vi "0MAIN _v2.vi"() -> ()   [LabVIEW 2014]
uses:
  <vilib>/Instr/_visa.llb/VISA Configure Serial Port (Instr).vi
  <vilib>/Instr/_visa.llb/VISA Open Access Mode.ctl
panel:
  out "OSL":bool
  out "Ошибка файла":errorcluster
  out "firstL":bool
  out "LN":bool
  out "WFL":bool
  out "SPL":bool
  out "umax":dbl
  out "umin":dbl
  out "fmax":dbl
  out "fmin":dbl
  out "FCD":bool
  out "LF2":bool
  out "LF1":bool
  out "В лог":string
  out "Строит":bool
  out "Ошибка temp":errorcluster
  out "Читает":bool
  out "Время старта":string
  out "Ошибка лога":errorcluster
  out "Файл данных":refnum<file>
  out "Файл журнала":refnum<file>
  in  "Управление":enum32{"Измерения", "График", "Настройки"}(tab)
  in  "SREP":bool
  in  "SR":bool
  in  "SP":T1 caption="Программа измерений" {"Шаг" format="%#_3g"; "Fкон" format="%#_3g"; "Fнач" format="%#_3g"}
  in  "Автограф":bool
  in  "Расчет графика":bool
  in  "TOF":bool
  in  "Частота метки 2":bool
  in  "Сохранение данных":bool
  in  "Очистка буфера":bool
  in  "Чтение данных":bool
  in  "Установить":string
  in  "Отправка":bool
  out "Данные с МК":string
  in  "Частота метки":bool
  in  "Выход":bool
  in  "Очистка массива":bool
  out "Сигналы":dbl[][](array[numeric]) caption="Сигнал Y, В" format="%#_3g"
  out "Метки":dbl[][](array[numeric]) caption="Метки:\nX (В)          Х (ГГц)"
  in  "SS":bool
  out "График":T2(graph)
  in  "Путь к файлу данных":path
  in  "Путь к логу":path
  in  "Логирование":bool
  out "Ошибка":T3
  in  "Порт":refnum<visa-resource-name>
  in  "Скорость передачи (9600)":u32=9600
  in  "Символ окончания (\\n)":u8=10 format="%.0x"
  in  "Режим доступа":T4 items=["VISA Defaults"=0, "Exclusive Lock"=1, "Load Configured Settings"=4]
  in  "Бит данных (8)":u8=8 format="%.0x"
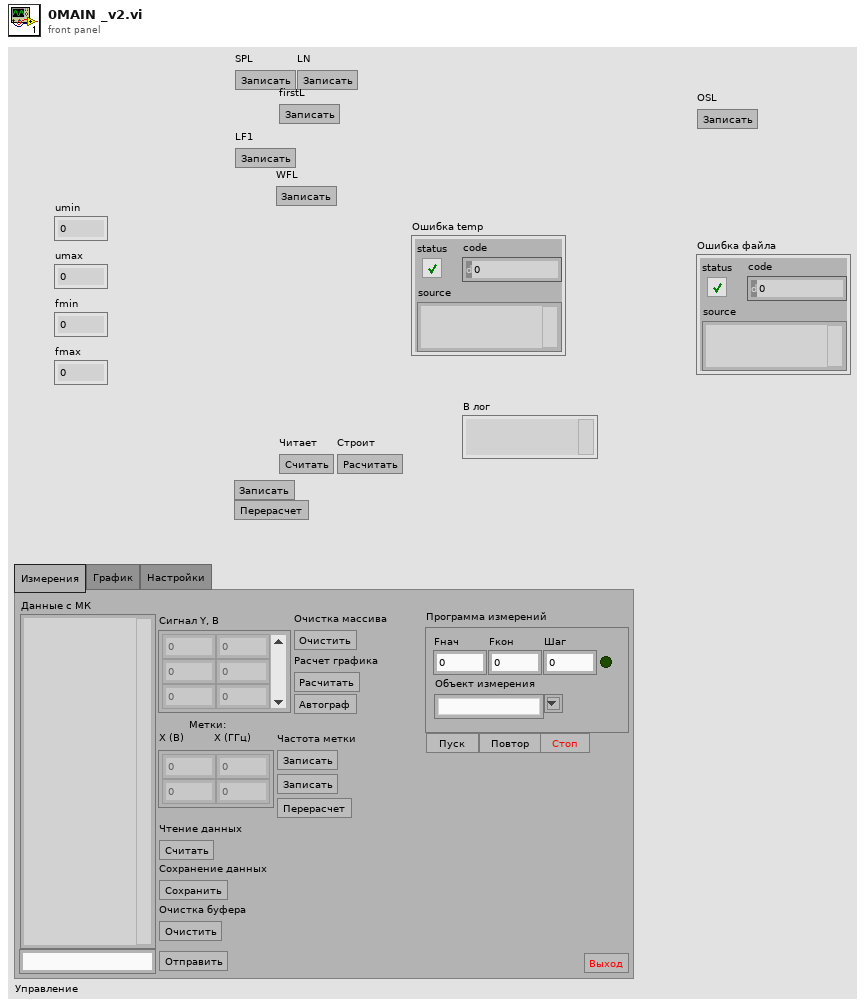
[diagram p1: front panel]
types:
  T1 = cluster{"Fнач":dbl, "Fкон":dbl, "Шаг":dbl, "ISR":bool, "ux":dbl, "i":u64, "n":u64, "MT":string}
  T2 = cluster{"Развертка X (В)":dbl[], "Сигнал Y (В)":dbl[]}
  T3 = cluster{"Статус":bool, "Код":i32, "Источник":string}
  T4 = typedef "VISA Open Access Mode.ctl" = u32
  T5 = enum16{"open", "replace", "create", "open or create", "replace or create", "replace or create with confirmation"}
  T6 = typedef "NI_Matrix.lvlib/RealMatrix.ctl" = dbl[][]
  T7 = enum32{"Измерения", "График", "Настройки", "Справка"}
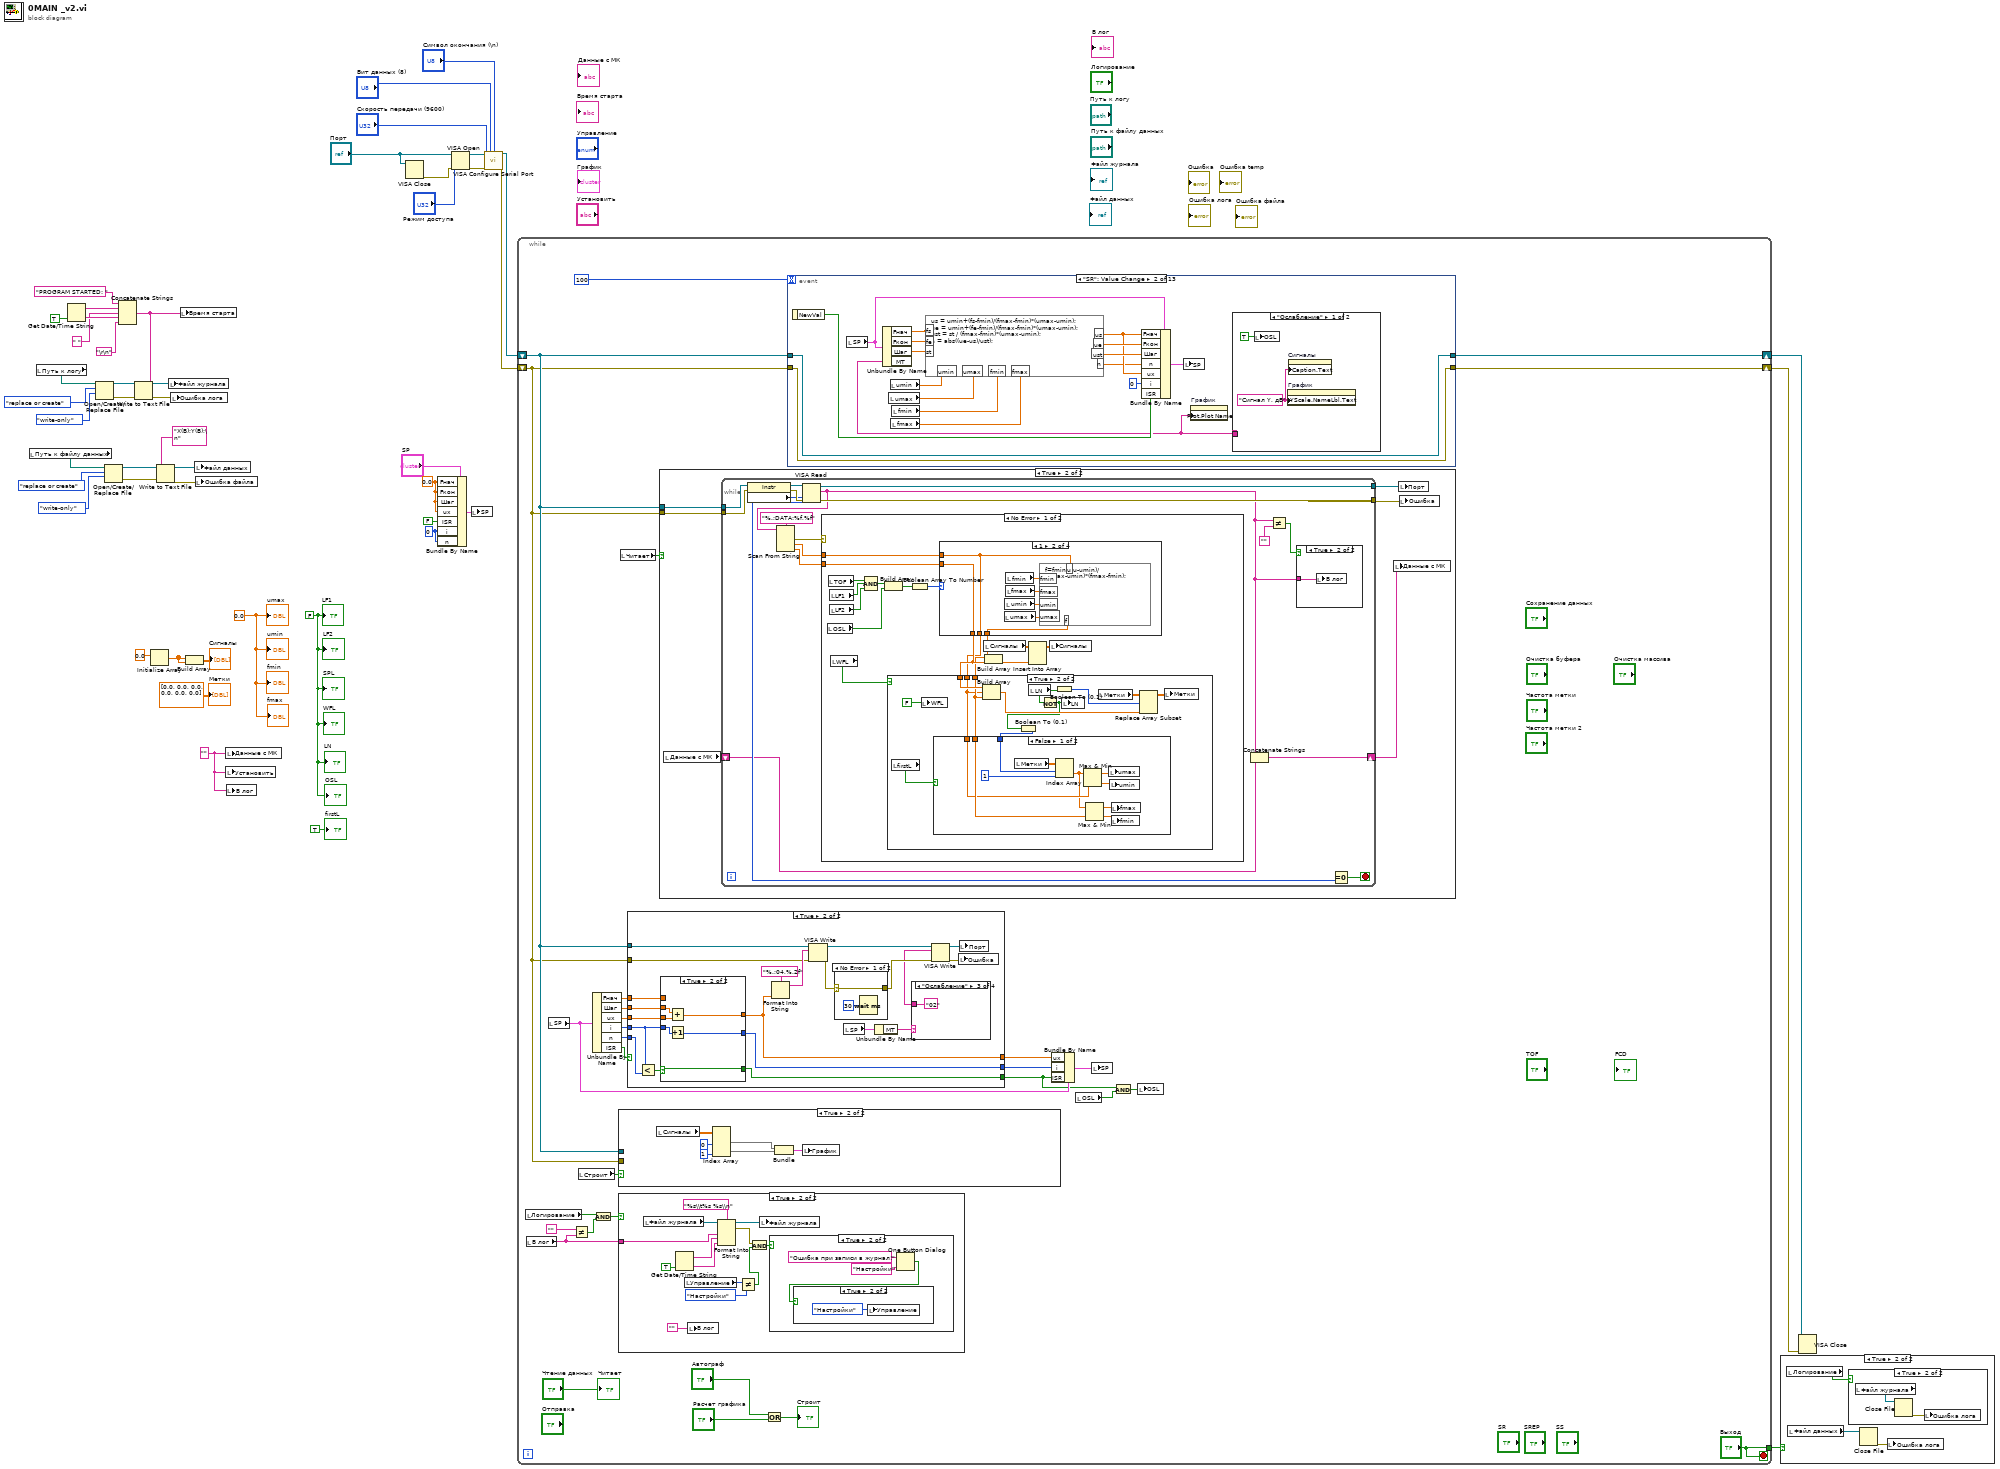
[diagram p0: block diagram]
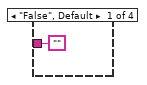
[diagram p5: hidden frame]
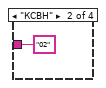
[diagram p6: hidden frame]
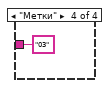
[diagram p7: hidden frame]
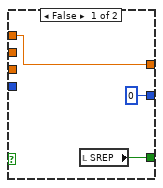
[diagram p9: hidden frame]
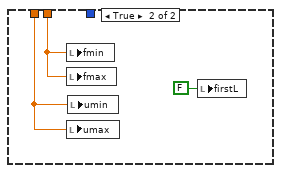
[diagram p17: hidden frame]
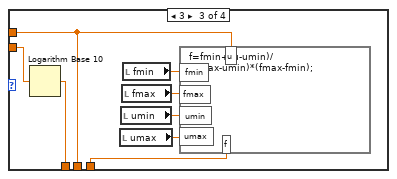
[diagram p19: hidden frame]
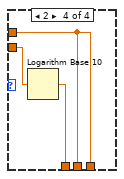
[diagram p20: hidden frame]
diagram:
  w12 = u64 0 ("i")
  w11 = 0.0 ("Fнач")
  w16 = 0.0 ("umax")
  w1 = FALSE ("LF1")
  w14 = "" ("Данные с МК")
  n1 = local read "Путь к файлу данных"() -> (w36:path)
  n2 = local read "Путь к логу"() -> (w4:path)
  n3 = Get Date/Time String(want seconds? (F)=TRUE) -> (date string=w32:string, time string=w24:string)  [unwired: 2 in]
  n4 = Open/Create/Replace File(file path (use dialog)=w4, operation (0:open)=T5."replace or create", access (0:read/write)=enum16{"read/write", "read-only", "write-only"}."write-only") -> (refnum out=w8:refnum<file>, error out=w7:errorcluster)  [unwired: 3 in, 1 out]
  n5 = Open/Create/Replace File(file path (use dialog)=w36, operation (0:open)=T5."replace or create", access (0:read/write)=enum16{"read/write", "read-only", "write-only"}."write-only") -> (refnum out=w26:refnum<file>, error out=w27:errorcluster)  [unwired: 3 in, 1 out]
  n6 = Concatenate Strings("PROGRAM STARTED: " ("string"), w32, " ", w24, "\r\n" ("string")) -> (w21:string)
  n7 = Write to Text File(file (use dialog)=w8, text=w21, error in=w7) -> (refnum out=w6:refnum<file>, error out=w5:errorcluster)  [unwired: 1 in, 1 out]
  n8 = Initialize Array(0.0 ("element")) -> (w17:dbl[])  [unwired: 1 in]
  n9 = Write to Text File(file (use dialog)=w26, text="X(В);Y(В);\n", error in=w27) -> (refnum out=w29:refnum<file>, error out=w30:errorcluster)  [unwired: 1 in, 1 out]
  n10 = local write "Файл журнала"(w6) -> ()
  n11 = local write "Ошибка лога"(w5) -> ()
  n12 = local write "Время старта"(w21) -> ()
  n13 = Build Array(w17, w17) -> (→"Сигналы":T6)
  n14 = local write "Файл данных"(w29) -> ()
  n15 = local write "Ошибка файла"(w30) -> ()
  n16 = local write "Данные с МК"(w14) -> ()
  n17 = local write "Установить"(w14) -> ()
  n18 = local write "В лог"(w14) -> ()
  n19 = VISA Close(VISA resource name="Порт") -> (error out=w37:errorcluster)  [unwired: 1 in]
  n20 = Bundle By Name(cluster="SP", "Fнач"=w11, "Fкон"=w11, "Шаг"=w11, "ux"=w11, "ISR"=FALSE, "i"=w12, "n"=w12) -> (w9:T1)
  n21 = VISA Open(access mode="Режим доступа", error in (no error)=w37, VISA resource name="Порт") -> (VISA resource name=w45:refnum<visa-resource-name>, error out=w44:errorcluster)  [unwired: 2 in]
  n22 = local write "SP"(w9) -> ()
  n23 = call-poly "VISA Configure Serial Port"("VISA resource name"=w45, "termination char\n(0xA = '\\n' = LF)"="Символ окончания (\\n)", "baud rate (9600)"="Скорость передачи (9600)", "data bits (8)"="Бит данных (8)", "error in (no error)"=w44) -> ("VISA resource name out"=w40:refnum<visa-resource-name>, "error out"=w42:errorcluster)  [unwired: 9 in]
  n24 = while {
    shift-right: [w78] -> w41
    shift-left: w42 -> [w53]
    shift-right: [w76] -> w39
    shift-left: w40 -> [w54]
    tunnel: ["Выход"] -> w22
    stop <- "Выход" stop-if-true
    n25 = local read "Логирование"() -> (w67:bool)
    n26 = local read "В лог"() -> (w64:string)
    n27 = local read "SP"() -> (w57:T1)
    n28 = Not Equal?(x="" ("y"), y=w64) -> (x != y?=w66:bool)
    n29 = local read "Строит"() -> (w70:bool)
    n30 = Unbundle By Name(w57) -> ("Fнач"=w59:dbl, "Шаг"=w60:dbl, "ux"=w61:dbl, "i"=w62:u64, "n"=w63:u64, "ISR"=w52:bool)
    n31 = And(x=w67, y=w66) -> (x .and. y?=w68:bool)
    n32 = case shown="True" w70 {
      tunnel: w53 -> [_ _]
      tunnel: w54 -> [_ _]
      frame False {
      }
      frame True {
        n33 = local read "Сигналы"() -> (w141:dbl[][])
        n34 = Index Array(array=w141, index (col) #1=0 ("disabled index (col)"), index (col) #2=1 ("index (col)")) -> (element #1=w138:dbl[], element #2=w136:dbl[])  [unwired: 2 in]
        n35 = Bundle("Сигналы"=w138, "Сигналы"=w136) -> (w137:cluster{"Сигналы":dbl[], "Сигналы":dbl[]})  [unwired: 1 in]
        n36 = local write "График"(w137) -> ()
      }
    }
    n37 = case shown="True" w68 {
      tunnel: w64 -> [_ w128]
      frame False {
      }
      frame True {
        n38 = local read "Файл журнала"() -> (w131:refnum<file>)
        n39 = Get Date/Time String(want seconds? (F)=TRUE) -> (date string=w127:string, time string=w126:string)  [unwired: 2 in]
        n40 = local read "Управление"() -> (w124:enum32{"Измерения", "График", "Настройки"})
        n41 = local write "В лог"("") -> ()
        n42 = Format Into String(format string="%s\\t%s %s\\n", initial string=w131, w128, w127, w126) -> (resulting string=w125:refnum<file>, error out=w122:errorcluster)  [unwired: 1 in]
        n43 = Not Equal?(x=w124, y=T7."Настройки" ("Управление")) -> (x != y?=w123:bool)
        n44 = And(x=w122, y=w123) -> (x .and. y?=w121:bool)
        n45 = local write "Файл журнала"(w125) -> ()
        n46 = case shown="True" w121 {
          frame False {
          }
          frame True {
            n47 = One Button Dialog(message="Ошибка при записи в журнал!", button name ("OK")="Настройки") -> (true=w132:bool)
            n48 = case shown="True" w132 {
              frame False {
              }
              frame True {
                n49 = local write "Управление"(T7."Настройки" ("Управление")) -> ()
              }
            }
          }
        }
      }
    }
    n50 = local read "Читает"() -> (w75:bool)
    n51 = case shown="True" w52 {
      selector: w52 -> [w81 _]
      tunnel: w63 -> [_ w102]
      tunnel: w62 -> [w80 w97]
      tunnel: w61 -> [w79 w99]
      tunnel: w60 -> [_ w98]
      tunnel: w59 -> [_ w95]
      tunnel: [w81 w100] -> w49
      tunnel: [w79 w90] -> w56
      tunnel: [w80 w96] -> w58
      tunnel: w54 -> [_ w88]
      tunnel: w53 -> [_ w87]
      frame False {
      }
      frame True {
        n52 = Less?(x=w97, y=w102) -> (x < y?=w101:bool)
        n53 = case shown="True" w101 {
          selector: w101 -> [_ w118]
          tunnel: [w111 w118] -> w100
          tunnel: w99 -> [_ w117]
          tunnel: w98 -> [_ w116]
          tunnel: w97 -> [_ w115]
          tunnel: [w112 w114] -> w90
          tunnel: [u64 0 w113] -> w96
          tunnel: w95 -> [w112 _]
          frame False {
            n54 = local read "SREP"() -> (w111:bool)
          }
          frame True {
            n55 = Add(x=w116, y=w117) -> (x+y=w114:dbl)
            n56 = Increment(x=w115) -> (x+1=w113:u64)
          }
        }
        n57 = Format Into String(format string="%.;04,%.2f", w90) -> (resulting string=w89:string)  [unwired: 2 in, 1 out]
        n58 = VISA Write(VISA resource name=w88, write buffer=w89, error in (no error)=w87) -> (VISA resource name out=w94:refnum<visa-resource-name>, error out=w93:errorcluster)  [unwired: 1 out]
        n59 = case shown="No Error" w93 {
          selector: w93 -> [w107 w109]
          tunnel: [w107 w109] -> w92
          frame No Error {
            n60 = Wait (ms)(milliseconds to wait=u32 30) -> ()  [unwired: 1 out]
          }
          frame Error {
          }
        }
        n61 = local read "SP"() -> (w84:T1)
        n62 = Unbundle By Name(w84) -> ("MT"=w83:string)
        n63 = case shown="\"Ослабление\"" w83 {
          tunnel: ["" "02" "02" "03"] -> w82
          frame "False", Default {
          }
          frame "КСВН" {
          }
          frame "Ослабление" {
          }
          frame "Метки" {
          }
        }
        n64 = VISA Write(VISA resource name=w94, write buffer=w82, error in (no error)=w92) -> (VISA resource name out=w86:refnum<visa-resource-name>, error out=w85:errorcluster)  [unwired: 1 out]
        n65 = local write "Ошибка"(w85) -> ()
        n66 = local write "Порт"(w86) -> ()
      }
    }
    n67 = case shown="True" w75 {
      tunnel: w53 -> [_ w146]
      tunnel: w54 -> [_ w147]
      frame False {
      }
      frame True {
        n68 = local read "Данные с МК"() -> (w145:string)
        n69 = while {
          tunnel: w147 -> [w160]
          tunnel: w146 -> [w159]
          shift-right: [w156] -> w142
          shift-left: w145 -> [w151]
          tunnel: [w158] -> w144
          tunnel: [w157] -> w143
          stop <- w155 stop-if-true
          n70 = property class="Instr"(reference=w160, error in=w159) -> (reference out=w164:refnum<visa-resource-name>, error out=w163:errorcluster, "Serial Settings:Number of Bytes at Serial Port"=w162:u32)
          n71 = VISA Read(VISA resource name=w164, byte count=w162, error in (no error)=w163) -> (VISA resource name out=w158:refnum<visa-resource-name>, read buffer=w148:string, error out=w157:errorcluster)  [unwired: 1 out]
          n72 = Scan From String(format string="%.;DATA:%f,%f", input string=w148) -> (error out=w154:errorcluster, output 1=w153:dbl, output 2=w152:dbl)  [unwired: 4 in, 2 out]
          n73 = case shown="No Error" w154 {
            tunnel: w153 -> [w177 _]
            tunnel: w152 -> [w178 _]
            frame No Error {
              n74 = local read "OSL"() -> (w168:bool)
              n75 = local read "TOF"() -> (w181:bool)
              n76 = local read "LF1"() -> (w180:bool)
              n77 = local read "LF2"() -> (w179:bool)
              n78 = local read "WFL"() -> (w173:bool)
              n79 = Compound Arithmetic op=AND(w181, w180, w179) -> (w169:bool)
              n80 = Build Array(w169, w168) -> (w166:bool[])
              n81 = Boolean Array To Number(Boolean array=w166) -> (number=w167:u32)
              n82 = case shown="1" w167 {
                tunnel: w178 -> [w208 w215 w217 w225]
                tunnel: w177 -> [w207 w214 w223 w226]
                tunnel: [w208 w215 w216 w224] -> w172
                tunnel: [w207 w214 w223 w226] -> w171
                tunnel: [w207 w213 w222 w226] -> w170
                frame 0, Default {
                }
                frame 1 {
                  n83 = local read "umax"() -> (w209:dbl)
                  n84 = local read "umin"() -> (w210:dbl)
                  n85 = local read "fmax"() -> (w211:dbl)
                  n86 = local read "fmin"() -> (w212:dbl)
                  n87 = formula code="f=fmin+(u-umin)/(umax-umin)*(fmax-fmin);"("fmin"=w212, "fmax"=w211, "umin"=w210, "umax"=w209, "u"=w214) -> ("f"=w213:dbl)
                }
                frame 3 {
                  n88 = Logarithm Base 10(1:w217) -> (0:w216:dbl)
                  n89 = local read "umax"() -> (w218:dbl)
                  n90 = local read "umin"() -> (w219:dbl)
                  n91 = local read "fmax"() -> (w220:dbl)
                  n92 = local read "fmin"() -> (w221:dbl)
                  n93 = formula code="f=fmin+(u-umin)/(umax-umin)*(fmax-fmin);"("fmin"=w221, "fmax"=w220, "umin"=w219, "umax"=w218, "u"=w223) -> ("f"=w222:dbl)
                }
                frame 2 {
                  n94 = Logarithm Base 10(1:w225) -> (0:w224:dbl)
                }
              }
              n95 = case shown="True" w173 {
                tunnel: w172 -> [_ w184]
                tunnel: w171 -> [_ w182]
                tunnel: w170 -> [_ w183]
                frame False {
                }
                frame True {
                  n96 = local read "firstL"() -> (w187:bool)
                  n97 = local write "WFL"(FALSE ("WFL")) -> ()
                  n98 = Build Array(w184, w182, w183) -> (w190:dbl[])
                  n99 = local read "LN"() -> (w188:bool)
                  n100 = Not(x=w188) -> (.not. x?=w186:bool)
                  n101 = Boolean To (0,1)(Boolean=w186) -> (0, 1=w185:i16)
                  n102 = case shown="False" w187 {
                    tunnel: w182 -> [w196 w205]
                    tunnel: w183 -> [w197 w206]
                    tunnel: w185 -> [w199 _]
                    frame False {
                      n103 = local read "Метки"() -> (w195:dbl[][])
                      n104 = Index Array(array=w195, index (row)=w199, index (col)=1) -> (element=w194:dbl)
                      n105 = Max & Min(x=w194, y=w196) -> (max(x,y)=w203:dbl, min(x,y)=w202:dbl)
                      n106 = Max & Min(x=w194, y=w197) -> (max(x,y)=w201:dbl, min(x,y)=w200:dbl)
                      n107 = local write "umax"(w203) -> ()
                      n108 = local write "umin"(w202) -> ()
                      n109 = local write "fmax"(w201) -> ()
                      n110 = local write "fmin"(w200) -> ()
                    }
                    frame True {
                      n111 = local write "fmin"(w206) -> ()
                      n112 = local write "fmax"(w206) -> ()
                      n113 = local write "umax"(w205) -> ()
                      n114 = local write "umin"(w205) -> ()
                      n115 = local write "firstL"(FALSE ("firstL")) -> ()
                    }
                  }
                  n116 = Boolean To (0,1)(Boolean=w188) -> (0, 1=w191:i16)
                  n117 = local write "LN"(w186) -> ()
                  n118 = local read "Метки"() -> (w193:dbl[][])
                  n119 = Replace Array Subset(array=w193, new element=w190, index (row)=w191) -> (w192:dbl[][])  [unwired: 1 in]
                  n120 = local write "Метки"(w192) -> ()
                }
              }
              n121 = local read "Сигналы"() -> (w176:dbl[][])
              n122 = Build Array(w170, w172) -> (w175:dbl[])
              n123 = Insert Into Array(array=w176, new element=w175) -> (w174:dbl[][])  [unwired: 2 in]
              n124 = local write "Сигналы"(w174) -> ()
            }
            frame Error {
            }
          }
          n125 = Concatenate Strings(w148, w151) -> (w156:string)
          n126 = Not Equal?(x=w148, y="") -> (x != y?=w149:bool)
          n127 = case shown="True" w149 {
            tunnel: w148 -> [_ w165]
            frame False {
            }
            frame True {
              n128 = local write "В лог"(w165) -> ()
            }
          }
          n129 = Equal To 0?(x=w162) -> (x = 0?=w155:bool)
        }
        n130 = local write "Данные с МК"(w142) -> ()
        n131 = local write "Порт"(w144) -> ()
        n132 = local write "Ошибка"(w143) -> ()
      }
    }
    n133 = Or(x="Автограф", y="Расчет графика") -> (x .or. y?=→"Строит":bool)
    n134 = event shown="[1] \"SR\": Value Change" {
      selector: _ -> [_ _ _ _ _ _ _ _ _ _ _ _ _]
      dyn-events: _ -> [_ _ _ _ _ _ _ _ _ _ _ _ _]
      timeout: 100 -> [_ _ _ _ _ _ _ _ _ _ _ _ _]
      tunnel: w54 -> [w228 w234 w257 w265 w309 w331 _ w381 w384 w390 w408 w428 w452]
      tunnel: w53 -> [w227 w235 w256 w264 w310 w332 w377 w380 w383 w391 w409 w429 w453]
      tunnel: [w228 w234 w257 w267 w309 w331 w369 w381 w384 w390 w408 w428 w452] -> w76
      tunnel: [w227 w235 w256 w266 w310 w332 w368 w380 w383 w391 w409 w429 w453] -> w78
      event Timeout {
        n135 = event-data() -> ()  [unwired: 1 in, 3 out]
      }
      event "SR": Value Change {
        n136 = event-data() -> ("NewVal"=w231:bool)  [unwired: 1 in]
        n137 = local read "SP"() -> (w246:T1)
        n138 = Unbundle By Name(w246) -> ("Fнач"=w244:dbl, "Fкон"=w243:dbl, "Шаг"=w242:dbl, "MT"=w229:string)
        n139 = local read "umax"() -> (w238:dbl)
        n140 = local read "umin"() -> (w239:dbl)
        n141 = local read "fmax"() -> (w236:dbl)
        n142 = local read "fmin"() -> (w237:dbl)
        n143 = formula code="us = umin+(fs-fmin)/(fmax-fmin)*(umax-umin);\nue = umin+(fe-fmin)/(fmax-fmin)*(umax-umin);\nust = st / (fmax-fmin)*(umax-umin);\nn = abs((ue-us)/ust);"("fs"=w244, "fe"=w243, "st"=w242, "umin"=w239, "umax"=w238, "fmin"=w237, "fmax"=w236) -> ("us"=w233:dbl, "ue"=w241:dbl, "ust"=w240:dbl, "n"=w232:dbl)
        n144 = Bundle By Name(cluster=w246, "Fнач"=w233, "Fкон"=w241, "Шаг"=w240, "n"=w232, "ux"=w233, "i"=u64 0, "ISR"=w231) -> (w245:T1)
        n145 = local write "SP"(w245) -> ()
        n146 = property on="График" class="XYGraph (strict)"("Plot.Plot Name"=w229) -> ()  [unwired: 2 in, 2 out]
        n147 = case shown="\"Ослабление\"" w229 {
          selector: w229 -> [w248 w251]
          tunnel: [w248 w251] -> _
          frame "Ослабление" {
            w247 = "Сигнал Y, дБ" ("Y Scale.Name Label.Text")
            n148 = local write "OSL"(TRUE ("OSL")) -> ()
            n149 = property on="График" class="XYGraph (strict)"("YScale.NameLbl.Text"=w247) -> ()  [unwired: 2 in, 2 out]
            n150 = property on="Сигналы" class="Arr (strict)"("Caption.Text"=w247) -> ()  [unwired: 2 in, 2 out]
          }
          frame Default {
            w250 = "Сигнал Y, В" ("Y Scale.Name Label.Text")
            n151 = local write "OSL"(FALSE ("OSL")) -> ()
            n152 = property on="График" class="XYGraph (strict)"("YScale.NameLbl.Text"=w250) -> ()  [unwired: 2 in, 2 out]
            n153 = property on="Сигналы" class="Arr (strict)"("Caption.Text"=w250) -> ()  [unwired: 2 in, 2 out]
          }
        }
      }
      event "SS": Value Change {
        n154 = event-data() -> ()  [unwired: 1 in, 1 out]
        n155 = local read "SP"() -> (w255:T1)
        n156 = Bundle By Name(cluster=w255, "ISR"=FALSE) -> (w253:T1)
        n157 = local write "SP"(w253) -> ()
      }
      event "Отправка": Value Change {
        n158 = event-data() -> ()  [unwired: 1 in, 1 out]
        n159 = local read "Установить"() -> (w259:string)
        n160 = Scan From String(format string="%d,%s", input string=w259) -> (error out=w262:errorcluster, output 1=w263:i32, output 2=w261:string)  [unwired: 4 in, 2 out]
        n161 = local write "Ошибка temp"(w262) -> ()
        n162 = case shown="3" w263 {
          tunnel: w261 -> [_ w273 _ _ w305]
          tunnel: ["" w269 "02" "03" w307] -> w258
          frame 0, Default {
          }
          frame 1 {
            n163 = local read "LF1"() -> (w271:bool)
            n164 = local read "LF2"() -> (w272:bool)
            n165 = And(x=w272, y=w271) -> (x .and. y?=w270:bool)
            n166 = case shown="True" w270 {
              tunnel: w273 -> [_ w287]
              tunnel: ["" w276] -> w269
              frame False {
                n167 = One Button Dialog(message="Ошибка!\nНе заданы частоты меток") -> ()  [unwired: 1 in, 1 out]
              }
              frame True {
                n168 = local read "umax"() -> (w277:dbl)
                n169 = local read "fmax"() -> (w279:dbl)
                n170 = local read "umin"() -> (w278:dbl)
                n171 = local read "fmin"() -> (w280:dbl)
                n172 = Scan From String(format string="%.;%f,%f", input string=w287) -> (output 1=w285:dbl, output 2=w284:dbl)  [unwired: 4 in, 3 out]
                n173 = formula code="u1 = umin + (f1 - fmin) / (fmax - fmin) * (umax - umin);\nu2 = umin + (f1 - fmin) / (fmax - fmin) * (umax - umin);"("f1"=w285, "f2"=w284, "fmin"=w280, "fmax"=w279, "umin"=w278, "umax"=w277) -> ("u1"=w282:dbl, "u2"=w281:dbl)
                n174 = Format Into String(format string="%.;01,%.2f,%.2f", w282, w281) -> (resulting string=w276:string)  [unwired: 2 in, 1 out]
              }
            }
          }
          frame 2 {
            n175 = local read "TOF"() -> (w289:bool)
            n176 = case shown="False" w289 {
              frame False {
                n177 = property on="График" class="XYGraph (strict)"("XScale.NameLbl.Text"="Развертка Х, В" ("X Scale.Name Label.Text")) -> ()  [unwired: 2 in, 2 out]
                n178 = property on="Сигналы" class="Arr (strict)"("Caption.Text"="           Сигналы:\nX (В)           Y (В)") -> ()  [unwired: 2 in, 2 out]
              }
              frame True {
              }
            }
            n179 = property on="График" class="XYGraph (strict)"("Plot.Plot Name"="КСВН") -> ()  [unwired: 2 in, 2 out]
          }
          frame 3 {
            w295 = TRUE ("SPL")
            n180 = local write "SPL"(w295) -> ()
            n181 = local write "WFL"(w295) -> ()
            n182 = property on="График" class="XYGraph (strict)"("Plot.Plot Name"="Метки") -> ()  [unwired: 2 in, 2 out]
            n183 = local read "TOF"() -> (w294:bool)
            n184 = case shown="True" w294 {
              frame False {
                n185 = property on="График" class="XYGraph (strict)"("XScale.NameLbl.Text"="Развертка Х, В" ("X Scale.Name Label.Text")) -> ()  [unwired: 2 in, 2 out]
                n186 = property on="Сигналы" class="Arr (strict)"("Caption.Text"="           Сигналы:\nX (В)           Y (В)") -> ()  [unwired: 2 in, 2 out]
              }
              frame True {
              }
            }
          }
          frame 4 {
            n187 = local read "umax"() -> (w303:dbl)
            n188 = local read "fmax"() -> (w301:dbl)
            n189 = local read "umin"() -> (w302:dbl)
            n190 = local read "fmin"() -> (w300:dbl)
            n191 = Scan From String(input string=w305) -> (error out=w306:errorcluster, output 1=w304:dbl)  [unwired: 4 in, 2 out]
            n192 = formula code="u = umin + (f - fmin) / (fmax - fmin) * (umax - umin);"("f"=w304, "fmin"=w300, "fmax"=w301, "umin"=w302, "umax"=w303) -> ("u"=w299:dbl)
            n193 = local write "Ошибка temp"(w306) -> ()
            n194 = Format Into String(format string="%.;04,%.2f", w299) -> (resulting string=w307:string)  [unwired: 2 in, 1 out]
          }
        }
        n195 = VISA Write(VISA resource name=w265, write buffer=w258, error in (no error)=w264) -> (VISA resource name out=w267:refnum<visa-resource-name>, error out=w266:errorcluster)  [unwired: 1 out]
      }
      event "Логирование": Value Change {
        n196 = event-data() -> ("NewVal"=w311:bool)  [unwired: 1 in]
        n197 = case shown="True" w311 {
          frame False {
          }
          frame True {
            n198 = local read "Путь к логу"() -> (w314:path)
            n199 = local read "Время старта"() -> (w317:string)
            n200 = Open/Create/Replace File(file path (use dialog)=w314, operation (0:open)=T5."replace or create", access (0:read/write)=enum16{"read/write", "read-only", "write-only"}."read/write") -> (refnum out=w319:refnum<file>, error out=w318:errorcluster)  [unwired: 3 in, 1 out]
            n201 = Format Into String(initial string=w319, error in=w318, w317) -> (resulting string=w316:refnum<file>, error out=w315:errorcluster)  [unwired: 1 in]
            n202 = local write "Файл журнала"(w316) -> ()
            n203 = local write "Ошибка лога"(w315) -> ()
          }
        }
        n204 = local read "Файл журнала"() -> (w313:refnum<file>)
        n205 = Close File(refnum=w313) -> (error out=w312:errorcluster)  [unwired: 1 in, 1 out]
        n206 = local write "Ошибка лога"(w312) -> ()
      }
      event "TOF": Value Change {
        n207 = event-data() -> ("NewVal"=w330:bool)  [unwired: 1 in]
        n208 = local read "umax"() -> (w326:dbl)
        n209 = local read "umin"() -> (w325:dbl)
        n210 = local read "fmax"() -> (w324:dbl)
        n211 = local read "fmin"() -> (w323:dbl)
        n212 = local read "Сигналы"() -> (w328:dbl[][])
        n213 = Matrix Size(0:w328) -> (1:w327:i32)  [unwired: 1 out]
        n214 = case shown="True" w330 {
          selector: w330 -> [w341 _]
          tunnel: [w341 w349] -> w322
          tunnel: w328 -> [w340 w348]
          tunnel: [w338 w347] -> w329
          tunnel: w327 -> [w339 w346]
          tunnel: w326 -> [w337 w342]
          tunnel: w325 -> [w336 w343]
          tunnel: w324 -> [w335 w344]
          tunnel: w323 -> [w334 w345]
          frame False {
            n215 = formula code="int i = 0;\nfor (i = 0; i < m; i+=1) {\n    S[i][0] = umin + (S[i][0] - fmin) / (fmax - fmin) * (umax - umin);\n}"("S"=w340, "m"=w339, "fmin"=w334, "fmax"=w335, "umin"=w336, "umax"=w337) -> ("S"=w338:dbl[][])
            n216 = property on="Сигналы" class="Arr (strict)"("Caption.Text"="           Сигналы:\nX (В)           Y (В)") -> ()  [unwired: 2 in, 2 out]
          }
          frame True {
            n217 = local read "LF1"() -> (w351:bool)
            n218 = local read "LF2"() -> (w352:bool)
            n219 = And(x=w351, y=w352) -> (x .and. y?=w350:bool)
            n220 = case shown="True" w350 {
              selector: w350 -> [w354 w365]
              tunnel: [w354 w365] -> w349
              tunnel: w348 -> [w353 w364]
              tunnel: [w353 w363] -> w347
              tunnel: w346 -> [_ w362]
              tunnel: w345 -> [_ w361]
              tunnel: w344 -> [_ w360]
              tunnel: w343 -> [_ w359]
              tunnel: w342 -> [_ w358]
              frame False {
                n221 = One Button Dialog(message="Ошибка!\nНе заданы частоты меток") -> ()  [unwired: 1 in, 1 out]
              }
              frame True {
                n222 = formula code="int i = 0;\nfor (i = 0; i < m; i+=1) {\n    S[i][0] = fmin + (S[i][0] - umin) / (umax - umin) * (fmax - fmin);\n}"("S"=w364, "m"=w362, "fmin"=w361, "fmax"=w360, "umin"=w359, "umax"=w358) -> ("S"=w363:dbl[][])
                n223 = property on="Сигналы" class="Arr (strict)"("Caption.Text"="           Сигналы:\nX (ГГц)           Y (В)") -> ()  [unwired: 2 in, 2 out]
                n224 = property on="График" class="XYGraph (strict)"("XScale.NameLbl.Text"="Частота Х, ГГц" ("X Scale.Name Label.Text")) -> ()  [unwired: 2 in, 2 out]
              }
            }
          }
        }
        n225 = local write "Сигналы"(w329) -> ()
        n226 = local write "FCD"(w322) -> ()
        n227 = local write "TOF"(w322) -> ()
      }
      event "Порт": Value Change {
        n228 = event-data() -> ("NewVal"=w376:refnum<visa-resource-name>, "OldVal"=w378:refnum<visa-resource-name>)  [unwired: 1 in]
        n229 = local read "Режим доступа"() -> (w375:T4)
        n230 = VISA Close(VISA resource name=w378, error in (no error)=w377) -> (error out=w366:errorcluster)
        n231 = local write "Ошибка temp"(w366) -> ()
        n232 = VISA Open(access mode=w375, VISA resource name=w376) -> (VISA resource name=w374:refnum<visa-resource-name>, error out=w373:errorcluster)  [unwired: 3 in]
        n233 = local read "Бит данных (8)"() -> (w371:u8)
        n234 = local read "Скорость передачи (9600)"() -> (w370:u32)
        n235 = local read "Символ окончания (\\n)"() -> (w372:u8)
        n236 = call-poly "VISA Configure Serial Port"("VISA resource name"=w374, "termination char\n(0xA = '\\n' = LF)"=w372, "baud rate (9600)"=w370, "data bits (8)"=w371, "error in (no error)"=w373) -> ("VISA resource name out"=w369:refnum<visa-resource-name>, "error out"=w368:errorcluster)  [unwired: 9 in]
        n237 = Wait (ms)(milliseconds to wait=u32 100) -> ()  [unwired: 1 out]
      }
      event "Очистка буфера": Value Change {
        n238 = event-data() -> ()  [unwired: 1 in, 1 out]
        n239 = local write "Данные с МК"("") -> ()
      }
      event "Очистка массива": Value Change {
        n240 = event-data() -> ()  [unwired: 1 in, 1 out]
        n241 = Initialize Array(0.0 ("element")) -> (w385:dbl[])  [unwired: 1 in]
        n242 = Build Array(w385, w385) -> (w382:T6)
        n243 = local write "Сигналы"(w382) -> ()
      }
      event "Частота метки 2": Value Change {
        n244 = event-data() -> ()  [unwired: 1 in, 1 out]
        n245 = local read "Установить"() -> (w387:string)
        n246 = Not Equal?(x=w387, y="") -> (x != y?=w388:bool)
        n247 = case shown="True" w388 {
          tunnel: w387 -> [_ w392]
          frame False {
          }
          frame True {
            w395 = TRUE ("LF1")
            n248 = local read "LF1"() -> (w396:bool)
            n249 = And(x=w395, y=w396) -> (x .and. y?=w394:bool)
            n250 = local write "LF2"(w395) -> ()
            n251 = Fract/Exp String To Number(string=w392) -> (number=w393:dbl)  [unwired: 3 in, 1 out]
            n252 = case shown="True" w394 {
              tunnel: w393 -> [_ w401]
              frame False {
              }
              frame True {
                n253 = local read "fmin"() -> (w402:dbl)
                n254 = Max & Min(x=w401, y=w402) -> (max(x,y)=w403:dbl, min(x,y)=w404:dbl)
                n255 = local write "fmax"(w403) -> ()
                n256 = local write "fmin"(w404) -> ()
              }
            }
            n257 = local read "Метки"() -> (w398:dbl[][])
            n258 = local write "fmax"(w393) -> ()
            n259 = Replace Array Subset(array=w398, new element=w393, index (row)=1 ("disabled index (row)"), index (col)=2 ("disabled index (col)")) -> (w397:T6)
            n260 = local write "Метки"(w397) -> ()
          }
        }
      }
      event "Частота метки": Value Change {
        n261 = event-data() -> ()  [unwired: 1 in, 1 out]
        n262 = local read "Установить"() -> (w406:string)
        n263 = Not Equal?(x=w406, y="") -> (x != y?=w407:bool)
        n264 = case shown="True" w407 {
          tunnel: w406 -> [_ w410]
          frame False {
          }
          frame True {
            w413 = TRUE ("LF1")
            n265 = local read "LF2"() -> (w414:bool)
            n266 = And(x=w413, y=w414) -> (x .and. y?=w412:bool)
            n267 = local write "LF1"(w413) -> ()
            n268 = Fract/Exp String To Number(string=w410) -> (number=w411:dbl)  [unwired: 3 in, 1 out]
            n269 = case shown="True" w412 {
              tunnel: w411 -> [_ w419]
              frame False {
              }
              frame True {
                n270 = local read "fmax"() -> (w420:dbl)
                n271 = Max & Min(x=w419, y=w420) -> (max(x,y)=w421:dbl, min(x,y)=w422:dbl)
                n272 = local write "fmax"(w421) -> ()
                n273 = local write "fmin"(w422) -> ()
              }
            }
            n274 = local read "Метки"() -> (w416:dbl[][])
            n275 = local write "fmin"(w411) -> ()
            n276 = Replace Array Subset(array=w416, new element=w411, index (row)=0 ("disabled index (row)"), index (col)=2 ("disabled index (col)")) -> (w415:T6)
            n277 = local write "Метки"(w415) -> ()
          }
        }
      }
      event "Сохранение данных": Value Change {
        n278 = event-data() -> ()  [unwired: 1 in, 1 out]
        n279 = while {
          shift-right: [w431] -> w425
          shift-left: _ -> [w430]
          i -> [w436]
          stop <- w435 stop-if-true
          n280 = local read "Сигналы"() -> (w438:dbl[][])
          n281 = Index Array(array=w438, index (row) #1=w436, index (col) #1=0 ("disabled index (col)"), index (row) #2=w436, index (col) #2=1 ("disabled index (col)")) -> (element #1=w434:dbl, element #2=w433:dbl)
          n282 = Format Into String(format string="%.;%f;%f\\n", initial string=w430, w434, w433) -> (resulting string=w431:string)  [unwired: 1 in, 1 out]
          n283 = Matrix Size(0:w438) -> (1:w437:i32)  [unwired: 1 out]
          n284 = Equal?(x=w436, y=w437) -> (x = y?=w435:bool)
        }
        n285 = local read "Файл данных"() -> (w427:refnum<file>)
        n286 = local read "Ошибка файла"() -> (w426:errorcluster)
        n287 = Write to Text File(file (use dialog)=w427, text=w425, error in=w426) -> (refnum out=w424:refnum<file>, error out=w423:errorcluster)  [unwired: 1 in, 1 out]
        n288 = local write "Ошибка файла"(w423) -> ()
        n289 = local write "Файл данных"(w424) -> ()
      }
      event "Путь к файлу данных": Value Change {
        n290 = event-data() -> ("NewVal"=w446:path)  [unwired: 1 in]
        n291 = local read "Файл данных"() -> (w451:refnum<file>)
        n292 = local read "Ошибка файла"() -> (w450:errorcluster)
        n293 = Close File(refnum=w451, error in=w450) -> (error out=w449:errorcluster)  [unwired: 1 out]
        n294 = local write "Ошибка файла"(w449) -> ()
        n295 = Open/Create/Replace File(file path (use dialog)=w446, operation (0:open)=T5."replace or create", access (0:read/write)=enum16{"read/write", "read-only", "write-only"}."write-only") -> (refnum out=w444:refnum<file>, error out=w445:errorcluster)  [unwired: 3 in, 1 out]
        n296 = Write to Text File(file (use dialog)=w444, text="X(В);Y(В);\n", error in=w445) -> (refnum out=w443:refnum<file>, error out=w442:errorcluster)  [unwired: 1 in, 1 out]
        n297 = local write "Ошибка файла"(w442) -> ()
        n298 = local write "Файл данных"(w443) -> ()
      }
    }
    n299 = Bundle By Name(cluster=w57, "ux"=w56, "i"=w58, "ISR"=w49) -> (w55:T1)
    n300 = local read "OSL"() -> (w50:bool)
    n301 = local write "SP"(w55) -> ()
    n302 = And(x=w49, y=w50) -> (x .and. y?=w51:bool)
    n303 = local write "OSL"(w51) -> ()
    "Читает" <- "Чтение данных"
  }
  n304 = case shown="True" w22 {
    frame False {
    }
    frame True {
      n305 = local read "Логирование"() -> (w456:bool)
      n306 = local read "Файл данных"() -> (w455:refnum<file>)
      n307 = case shown="True" w456 {
        frame False {
        }
        frame True {
          n308 = local read "Файл журнала"() -> (w458:refnum<file>)
          n309 = Close File(refnum=w458) -> (error out=w457:errorcluster)  [unwired: 1 in, 1 out]
          n310 = local write "Ошибка лога"(w457) -> ()
        }
      }
      n311 = Close File(refnum=w455) -> (error out=w454:errorcluster)  [unwired: 1 in, 1 out]
      n312 = local write "Ошибка лога"(w454) -> ()
    }
  }
  n313 = VISA Close(VISA resource name=w39, error in (no error)=w41) -> ()  [unwired: 1 out]
  "Метки" <- dbl[][] [[0.0, 0.0, 0.0], [0.0, 0.0, 0.0]] ("Метки")
  "fmin" <- w16
  "fmax" <- w16
  "umin" <- w16
  "umax" <- w16
  "LF1" <- w1
  "LF2" <- w1
  "SPL" <- w1
  "WFL" <- w1
  "LN" <- w1
  "firstL" <- TRUE ("firstL")
  "OSL" <- w1
